vi "Degrees to Array Length.vi"(11 "Degrees":i32) -> (3 "Array Length":i8)   [LabVIEW 2016]
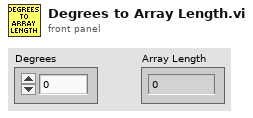
[diagram p1: front panel]
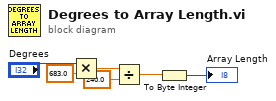
[diagram p0: block diagram]
diagram:
  n1 = Multiply(x="Degrees", y=683.0) -> (x*y=w4:dbl)
  n2 = Divide(x=w4, y=240.0) -> (x/y=w2:dbl)
  n3 = To Byte Integer(number=w2) -> (8bit integer=→"Array Length":i8)
